vi "FaultClear.vi"(10 "Channel":string) -> (0 "error out":errorcluster, 2 "Channel out":string)   [LabVIEW 2015, in "ni-veristand-steps-runtime-lib.lvlib"]
uses:
  ni-veristand-steps-runtime-lib.lvlib
  <vilib>/NI Veristand/Execution/ChannelFaultManager/NI_VS ChannelFault ExecutionAPI.lvlib
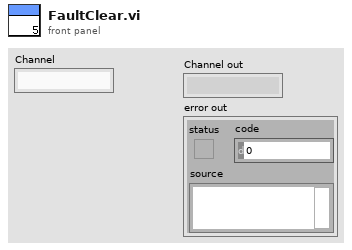
[diagram p1: front panel]
types:
  T1 = typedef "ni-veristand-steps-runtime-lib.lvlib/VeriStand dotNet References.ctl" = cluster{"Project Ref":refnum<k24>, "Workspace Manager Ref":refnum<k24>, "Model Manager Ref":refnum<k24>, "Channel Fault Manager Ref":refnum<k24>}
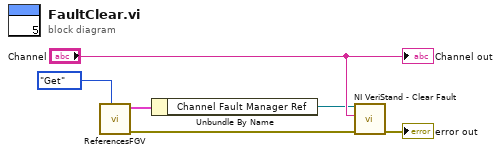
[diagram p0: block diagram]
diagram:
  n1 = call "ReferencesFGV.vi"("Get/Set"=enum16{"Get", "Set"}."Get") -> ("error out"=w4:errorcluster, "VeriStand dotNET Refs out"=w2:T1)  [unwired: 9 in]
  n2 = Unbundle By Name(w2) -> ("Channel Fault Manager Ref"=w1:refnum<k24>)
  n3 = call <vilib>:"NI VeriStand - Clear Fault.vi"("error in (no error)"=w4, "Channel"="Channel", "ChannelFault in"=w1) -> ("error out"=→"error out":errorcluster)  [unwired: 7 in, 1 out]
  "Channel out" <- "Channel"
